vi "Read Set Shed Sequence Status.vi"(11 "Set Shed Sequence Status Msg in":refnum<class "Set Shed Sequence Status Msg.lvclass">) -> (0 "Status":T1, 1 "error":string, 2 "Sequence":string, 3 "Set Shed Sequence Status Msg out":refnum<class "Set Shed Sequence Status Msg.lvclass">)   [LabVIEW 2015, in "SCADA Core.lvlib" / "Set Shed Sequence Status Msg.lvclass"]
uses:
  Set Shed Sequence Status Msg.lvclass
  Set Shed Sequence Status.ctl
  Set Shed Sequence Status Msg.lvclass/Set Shed Sequence Status Msg.ctl
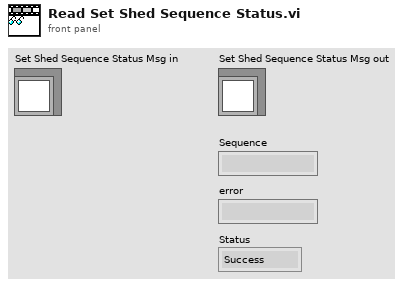
[diagram p1: front panel]
types:
  T1 = typedef "SCADA Core.lvlib/Set Shed Sequence Status Msg.lvclass/Set Shed Sequence Status.ctl" = enum16{"Success", "Failure"}
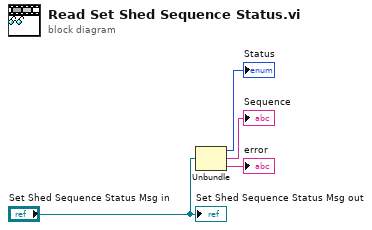
[diagram p0: block diagram]
diagram:
  n1 = Unbundle("Set Shed Sequence Status Msg in") -> (→"Status":T1, →"Sequence":string, →"error":string)
  "Set Shed Sequence Status Msg out" <- "Set Shed Sequence Status Msg in"
